vi "PulsePrams.vi"(4 "sample rate (s/Pt)":dbl format="%.2f", 5 "Compute window?":bool, 6 "Length of Subset":i32, 7 "Pressure Cal Parameters":T1={"Center Freq (MHz)"=0.0, "PRF (kHz)"=0.0, "Pulse window (us)"=0.0, "Hydrophone"=enum."PAL #1048", "booster amp?"=TRUE} {"Pulse window (us)" format="%.2f"; "PRF (kHz)" format="%.2f"; "Center Freq (MHz)" format="%.2f"}, 8 "Index of subset":i32, 9 "delay (ms)":dbl format="%.2f", 11 "Data":dbl[](array[numeric]) format="%.2f") -> (3 "Pulse Parameters":T3 {"pos peak pressure (MPa)" format="%.2f"; "focal length (cm)" format="%.2f"; "MI" format="%.2f"; "Ita.3" format="%.2f"; "Temporal Av Intensity \n(Ita mW/cm^2)" format="%.2f"; "Ipa.3" format="%.2f"; "Pulse Av Intensity\n (Ipa W/cm^2)" format="%.2f"; "Pulse Int \nIntegral (PII J/cm^2)" format="%.4e"; "pulse dur (Pd s)" format="%.2e"; "p.3" format="%.2f"; "neg peak pressure (MPa)" format="%.2f"; "derating (.3) factor" format="%.2f"; "prf" format="%.2f"; "Frequency (MHz)" format="%.2f"})   [LabVIEW 2022 SP3]
uses:
  HydrophoneSettings.ctl
  Hydros.ctl
  ScanningControl/Pulsers/PulserGlobals.vi
  Patient Routines/PatientGlobals.vi
panel:
  out "Waveform Graph":dbl[](graph)
  # "If true then calculate the index and number of points to extract pulse"
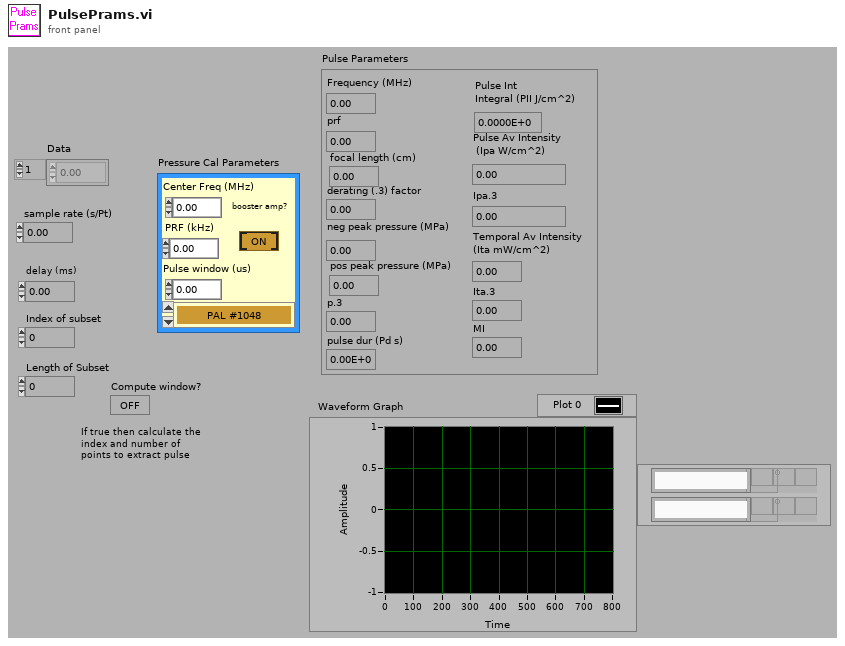
[diagram p1: front panel]
types:
  T1 = typedef "HydrophoneSettings.ctl" = cluster{"Center Freq (MHz)":dbl, "PRF (kHz)":dbl, "Pulse window (us)":dbl, "Hydrophone":T2, "booster amp?":bool}
  T2 = typedef "Hydros.ctl" = enum16{"PAL #1048", "PAL #525", "PAL #430a", "PAL #192", "DEAD PAL # 1403", "LOST UHI Onda", "DEAD PAL #1818", "PAL #1974", "DEAD #2266 w/booster", "PAL #2524 w/booster", "PAL FP21-20T", "PAL FP160-13  ", "PAL FP141-20", "PAL FP158-08T"}
  T3 = cluster{"Frequency (MHz)":dbl, "prf":dbl, "focal length (cm)":dbl, "derating (.3) factor":dbl, "neg peak pressure (MPa)":dbl, "pos peak pressure (MPa)":dbl, "p.3":dbl, "pulse dur (Pd s)":dbl, "Pulse Int \nIntegral (PII J/cm^2)":dbl, "Pulse Av Intensity\n (Ipa W/cm^2)":dbl, "Ipa.3":dbl, "Temporal Av Intensity \n(Ita mW/cm^2)":dbl, "Ita.3":dbl, "MI":dbl}
  T4 = cluster{"Therapy frequency (MHz)":dbl, "Therapy amplitude (mV)":dbl, "time therapy on (s)":dbl, "Therapy Delay (ms) ":dbl, "Time (s)":dbl}
  T5 = typedef "PatientInfoDef.ctl" = cluster{"Eye Selector":enum32{"Left", "Right"}, "Plane":i8, "First Name":string, "Last Name":string, "Notes":string, "Patient ID":string, "Scan Location":enum32{"Radio Selection 1", "Radio Selection 2"}}
  T6 = cluster{"pulse dur (Pd s)":dbl, "Temporal Av Intensity \n(Ita mW/cm^2)":dbl, "Pulse Av Intensity\n (Ipa W/cm^2)":dbl, "Pulse Int \nIntegral (PII J/cm^2)":dbl}
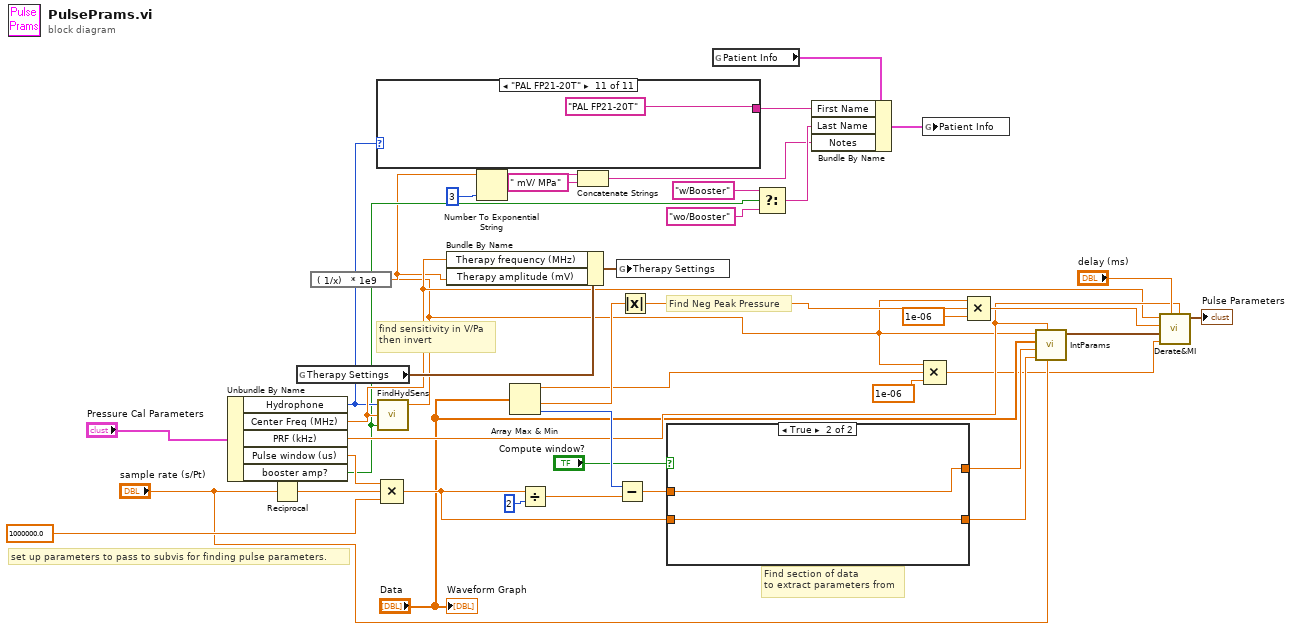
[diagram p0: block diagram]
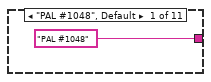
[diagram p2: hidden frame]
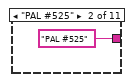
[diagram p3: hidden frame]
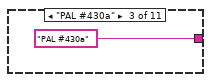
[diagram p4: hidden frame]
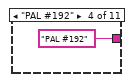
[diagram p5: hidden frame]
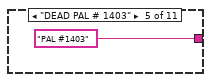
[diagram p6: hidden frame]
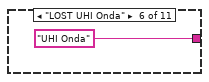
[diagram p7: hidden frame]
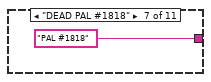
[diagram p8: hidden frame]
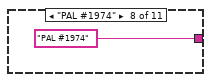
[diagram p9: hidden frame]
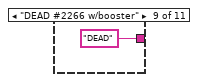
[diagram p10: hidden frame]
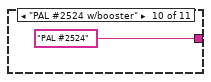
[diagram p11: hidden frame]
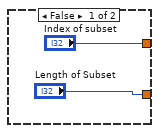
[diagram p12: hidden frame]
diagram:
  # "set up parameters to pass to subvis for finding pulse parameters."
  # "Find section of data\nto extract parameters from"
  # "Find Neg Peak Pressure"
  # "find sensitivity in V/Pa\nthen invert"
  n1 = Unbundle By Name("Pressure Cal Parameters") -> ("Hydrophone"=w17:T2, "Center Freq (MHz)"=w18:dbl, "PRF (kHz)"=w22:dbl, "Pulse window (us)"=w30:dbl, "booster amp?"=w7:bool)
  n2 = Reciprocal(x="sample rate (s/Pt)") -> (1/x=w33:dbl)
  n3 = global read "PulserGlobals.vi" "Therapy Settings"() -> (w20:T4)
  n4 = case shown="\"PAL FP21-20T\"" w17 {
    tunnel: ["PAL #1048" ("Patient ID") "PAL #525" ("Patient ID") "PAL #430a" ("Patient ID") "PAL #192" ("Patient ID") "PAL #1403" ("Patient ID") "UHI Onda" ("Patient ID") "PAL #1818" ("Patient ID") "PAL #1974" ("Patient ID") "DEAD" ("Patient ID") "PAL #2524" ("Patient ID") "PAL FP21-20T" ("Patient ID")] -> w14
    frame "PAL #1048", Default {
    }
    frame "PAL #525" {
    }
    frame "PAL #430a" {
    }
    frame "PAL #192" {
    }
    frame "DEAD PAL # 1403" {
    }
    frame "LOST UHI Onda" {
    }
    frame "DEAD PAL #1818" {
    }
    frame "PAL #1974" {
    }
    frame "DEAD #2266 w/booster" {
    }
    frame "PAL #2524 w/booster" {
    }
    frame "PAL FP21-20T" {
    }
  }
  n5 = call "FindHydSens.vi"("booster amp?"=w7, "Frequency (MHz)"=w18, "Hydrophone"=w17) -> ("Sensitivity in Pa/V"=w3:dbl)  [unwired: 2 out]
  n6 = expression code="( 1/x)   * 1e9"(w3) -> (w6:dbl)
  n7 = Compound Arithmetic op=MULTIPLY(w30, w33, 1000000.0 ("x")) -> (w27:dbl)
  n8 = Bundle By Name(cluster=w20, "Therapy frequency (MHz)"=w18, "Therapy amplitude (mV)"=w6) -> (w19:T4)
  n9 = Number To Exponential String(number=w6, precision (6)=i16 3 ("width (-)")) -> (E-format string=w10:string)  [unwired: 2 in]
  n10 = Array Max & Min(array="Data") -> (max value=w2:dbl, min value=w41:dbl, min index (indices)=w35:i32)  [unwired: 1 out]
  n11 = Divide(x=w27, y=2) -> (x/y=w34:dbl)
  n12 = Concatenate Strings(w10, " mV/ MPa" ("string")) -> (w9:string)
  n13 = global write "PulserGlobals.vi" "Therapy Settings"(w19) -> ()
  n14 = Subtract(x=w35, y=w34) -> (x-y=w28:dbl)
  n15 = Absolute Value(x=w41) -> (abs(x)=w23:dbl)
  n16 = case shown="True" "Compute window?" {
    tunnel: w28 -> [_ w57]
    tunnel: ["Index of subset" w57] -> w25
    tunnel: ["Length of Subset" w56] -> w26
    tunnel: w27 -> [_ w56]
    frame False {
    }
    frame True {
    }
  }
  n17 = global read "PatientGlobals.vi" "Patient Info"() -> (w16:T5)
  n18 = Select(t="w/Booster" ("Last Name"), s=w7, f="wo/Booster") -> (s? t:f=w13:string)
  n19 = Bundle By Name(cluster=w16, "First Name"=w14, "Last Name"=w13, "Notes"=w9) -> (w15:T5)
  n20 = global write "PatientGlobals.vi" "Patient Info"(w15) -> ()
  n21 = Compound Arithmetic op=MULTIPLY(w3, w2, 1e-06 ("x")) -> (w1:dbl)
  n22 = Compound Arithmetic op=MULTIPLY(w3, w23, 1e-06 ("x")) -> (w40:dbl)
  n23 = call "IntParams.vi"("sample interval (s/Pt)"="sample rate (s/Pt)", "prf"=w22, "Length of Subset"=w26, "Index of subset"=w25, "Data"="Data", "Sens"=w3) -> ("Intensity Variables"=w38:T6)  [unwired: 1 in, 4 out]
  n24 = call "Derate&MI.vi"("Frequency (MHz)"=w18, "neg peak pressure (MPa)"=w40, "Intensity Variables"=w38, "pos peak pressure (MPa)"=w1, "delay (ms)"="delay (ms)", "prf"=w22) -> ("Pulse Parameters"=→"Pulse Parameters":T3)  [unwired: 4 out]
  "Waveform Graph" <- "Data"
